vi "Init Test WAMP.vi"(8 "error in":errorcluster, 10 "Address":string="ws://localhost:8080/", 11 "Realm":string="default_realm") -> (0 "error out":errorcluster, 3 "wamplv.lvlib:Test WAMP":refnum<class "Test WAMP.lvclass">)   [LabVIEW 2021, in "Test WAMP.lvclass"]
uses:
  Test WAMP.lvclass
  Test WAMP.lvclass/Test WAMP.ctl
  <vilib>/LabVIEW Open Source Project/OpenURI/uri/URI.lvclass
  <vilib>/Utility/error.llb/Error Cluster From Error Code.vi
  <vilib>/ErrorRing/Error Ring.xnode
  Private/Comm Handlers/RawSocket TCP Handler/RawSocket TCP Handler.lvclass
  WAMP Client/API/TypeDefs/Transport Type.ctl
  WAMP Client/WAMP Client.lvclass
  Private/Comm Handlers/Websocket Handler/Websocket Handler.lvclass
  D:/Git/wamplv/Private/Comm Handlers/TCPSocketBasedCommHandlerBase/TCPSocketBasedCommHandlerBase.lvclass
  D:/Git/wamplv/Private/Comm Handlers/CommHandlerBase/CommHandlerBase.lvclass
  D:/Git/wamplv/Private/Comm Handlers/ICommHandler/ICommHandler.lvclass
  D:/Git/wamplv/Private/Comm Handlers/RawSocket TCP Handler/RawSocket TCP Handler.lvclass
  D:/Git/wamplv/Private/Comm Handlers/Websocket Handler/Websocket Handler.lvclass
  Private/Comm Handlers/TCPSocketBasedCommHandlerBase/TCPSocketBasedCommHandlerBase.lvclass
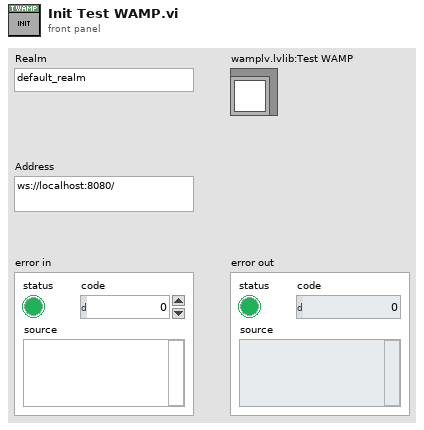
[diagram p1: front panel]
types:
  T1 = typedef "wamplv.lvlib/WAMP Client.lvclass/Transport Type.ctl" = enum16{"WebSocket", "RawSocket TCP"}
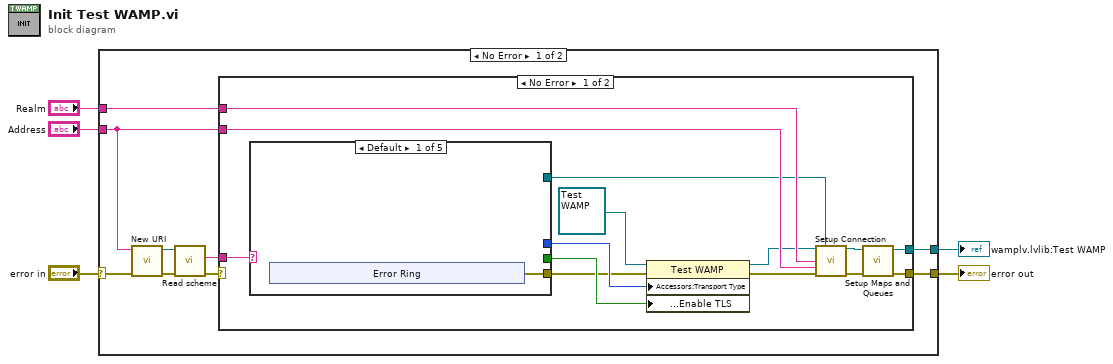
[diagram p0: block diagram]
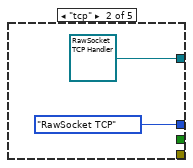
[diagram p2: hidden frame]
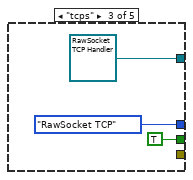
[diagram p3: hidden frame]
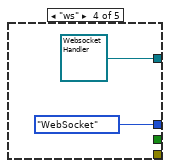
[diagram p4: hidden frame]
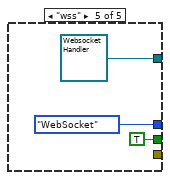
[diagram p5: hidden frame]
diagram:
  n1 = case shown="No Error" "error in" {
    selector: "error in" -> [w10 w45]
    tunnel: [w6 w45] -> w4
    tunnel: [w7 _] -> w3
    tunnel: "Address" -> [w9 _]
    tunnel: "Realm" -> [w8 _]
    frame No Error {
      n2 = call <vilib>:"New URI.vi"("error in (no error)"=w10, "URI"=w9) -> ("error out"=w12:errorcluster, "URI"=w11:refnum<class "URI.lvclass">)  [unwired: 8 in]
      n3 = call <vilib>:"Read scheme.vi"("error in (no error)"=w12, "URI in"=w11) -> ("error out"=w13:errorcluster, "scheme"=w14:string)  [unwired: 7 in, 1 out]
      n4 = case shown="No Error" w13 {
        selector: w13 -> [_ w44]
        tunnel: w8 -> [w28 _]
        tunnel: [w27 _] -> w7
        tunnel: [w26 w44] -> w6
        tunnel: w9 -> [w25 _]
        tunnel: w14 -> [w24 _]
        frame No Error {
          n5 = case shown="Default" w24 {
            tunnel: [_ refnum<class "RawSocket TCP Handler.lvclass"> refnum ("wamplv.lvlib:RawSocket Handler.lvclass") refnum<class "RawSocket TCP Handler.lvclass"> refnum ("wamplv.lvlib:RawSocket Handler.lvclass") refnum<class "Websocket Handler.lvclass"> refnum ("Websocket Handler.lvclass") refnum<class "Websocket Handler.lvclass"> refnum ("Websocket Handler.lvclass")] -> w23
            tunnel: [w29 _ _ _ _] -> w17
            tunnel: [_ Transport_Type."RawSocket TCP" ("Transport Type") Transport_Type."RawSocket TCP" ("Transport Type") Transport_Type."WebSocket" ("Transport Type") Transport_Type."WebSocket" ("Transport Type")] -> w19
            tunnel: [_ _ TRUE ("Transport Options.Enable TLS?") _ TRUE ("Transport Options.Enable TLS?")] -> w18
            frame Default {
              n6 = xnode "Error Ring"() -> ("error out"=w29:errorcluster)
            }
            frame "tcp" {
            }
            frame "tcps" {
            }
            frame "ws" {
            }
            frame "wss" {
            }
          }
          n7 = property class="Test WAMP"(reference=refnum<class "Test WAMP.lvclass"> refnum ("wamplv.lvlib:Test WAMP"), error in=w17, "Accessors:Transport Type "=w19, "Accessors:Transport Settings:Enable TLS"=w18) -> (reference out=w20:refnum<class "Test WAMP.lvclass">, error out=w16:errorcluster)
          n8 = call-dynamic "Setup Connection.vi"("WAMP Client in"=w20, "ICommHandler.lvclass"=w23, "Realm"=w28, "Address"=w25, "error in (no error)"=w16) -> ("WAMP Client out"=w22:refnum<class "Test WAMP.lvclass">, "error out"=w21:errorcluster)  [unwired: 9 in]
          n9 = call-dynamic "Setup Maps and Queues.vi"("error in (no error)"=w21, "WAMP Client in"=w22) -> ("error out"=w26:errorcluster, "WAMP Client out"=w27:refnum<class "Test WAMP.lvclass">)  [unwired: 8 in]
        }
        frame Error {
        }
      }
    }
    frame Error {
    }
  }
  "error out" <- w4
  "wamplv.lvlib:Test WAMP" <- w3
